vi "correct slipping wheels.vi"(7 "deslizamento?":bool, 10 "Matriz m \nesperada":T1, 11 "Matriz m\nobservada":T1) -> (2 "m sem \ndeslizamento \ne no \nsentido \noriginal":dbl[](array[numeric]), 3 "m sem\ndeslizamento":T1)   [LabVIEW 2018]
uses:
  <vilib>/Analysis/Matrix/Datatypes/RealMatrix.ctl
  <vilib>/Analysis/Matrix/Numeric/Subtract/Subtract - RM,RM.vi
  <vilib>/Analysis/Matrix/NI_Matrix.lvlib
panel:
  out "<f,m_o>/|f|^2":dbl format="%.2f"
  out "error":i32
  out "error 2":i32
  out "<m_o,m_c>":dbl format="%.2f"
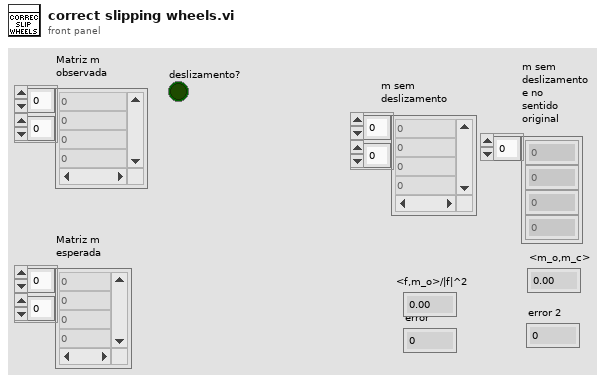
[diagram p1: front panel]
types:
  T1 = typedef "NI_Matrix.lvlib/RealMatrix.ctl" = dbl[][]
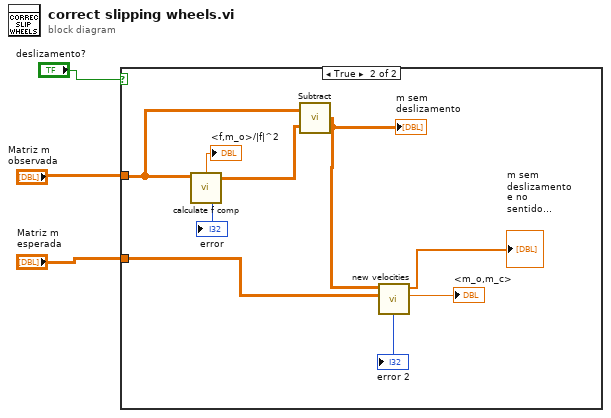
[diagram p0: block diagram]
diagram:
  n1 = case shown="True" "deslizamento?" {
    tunnel: "Matriz m\nobservada" -> [_ w12]
    tunnel: "Matriz m \nesperada" -> [_ w7]
    frame False {
    }
    frame True {
      n2 = call "calculate f comp.vi"("Matriz m\nobservada"=w12) -> ("Componente \nde n_o em f"=w11:T1, "<f,m_o>/|f|^2"=→"<f,m_o>/|f|^2":dbl, "error"=→"error":i32)  [unwired: 8 in]
      n3 = call-poly <vilib>:"Subtract.vi"("Real Matrix B"=w11, "Real Matrix A"=w12) -> ("A - B"=w8:T1)
      "m sem\ndeslizamento" <- w8
      n4 = call "new velocities.vi"("Matriz m \nesperada"=w7, "m sem\ndeslizamento"=w8) -> ("<m_o,m_c>"=→"<m_o,m_c>":dbl, "m sem \ndeslizamento \ne no \nsentido \noriginal"=→"m sem \ndeslizamento \ne no \nsentido \noriginal":dbl[], "error"=→"error 2":i32)  [unwired: 7 in]
    }
  }
